vi "Curtin1_GlobalFolder.vi"() -> (1 "LabVIEW Data Path":path, 2 "Samples":path)   [LabVIEW 2022 SP3]
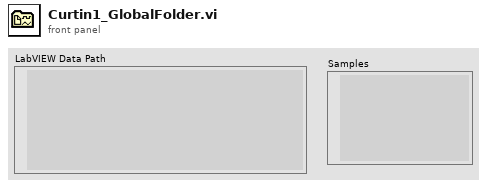
[diagram p1: front panel]
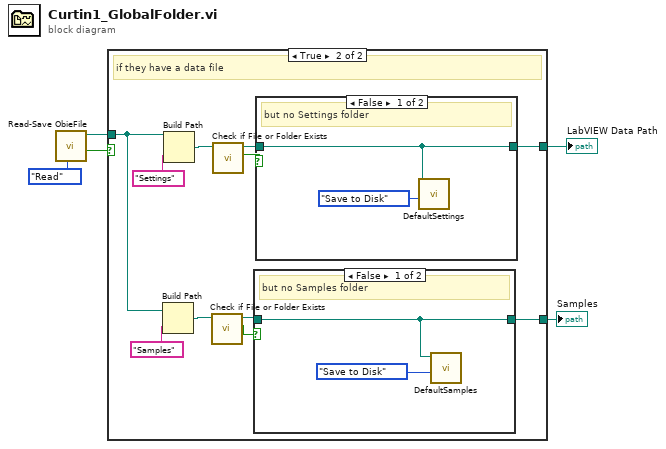
[diagram p0: block diagram]
diagram:
  n1 = call "Read-Save ObieFile.vi"("Task"=enum16{"Save", "Read"}."Read") -> ("Success?"=w2:bool, "DataPath Out"=w3:path)  [unwired: 8 in, 1 out]
  n2 = case shown="True" w2 {
    tunnel: [w6 w13] -> w5
    tunnel: w3 -> [w6 w10]
    tunnel: [w6 w7] -> w1
    frame False {
      # "they have not set up the data folder yet"
    }
    frame True {
      # "if they have a data file"
      n3 = Build Path(base path=w10, name or relative path="Samples") -> (appended path=w12:path)
      n4 = Build Path(base path=w10, name or relative path="Settings") -> (appended path=w14:path)
      n5 = call <vilib>:"Check if File or Folder Exists.vi"("path"=w12) -> ("file or folder exists?"=w8:bool, "dup path"=w9:path)  [unwired: 8 in, 1 out]
      n6 = call <vilib>:"Check if File or Folder Exists.vi"("path"=w14) -> ("file or folder exists?"=w16:bool, "dup path"=w15:path)  [unwired: 8 in, 1 out]
      n7 = case shown="False" w8 {
        tunnel: [w19 w20] -> w7
        tunnel: w9 -> [w19 w20]
        frame False {
          # "but no Samples folder"
          n8 = call "DefaultSamples.vi"("Task"=enum16{"Load to VI", "Save to Disk"}."Save to Disk", "path (use dialog)"=w19) -> ()  [unwired: 9 in, 1 out]
        }
        frame True {
          # "and a settings folder"
        }
      }
      n9 = case shown="False" w16 {
        tunnel: [w21 w23] -> w13
        tunnel: w15 -> [w21 w23]
        frame False {
          # "but no Settings folder"
          n10 = call "DefaultSettings.vi"("Task"=enum16{"Load to VI", "Save to Disk"}."Save to Disk", "path (use dialog)"=w21) -> ()  [unwired: 9 in, 1 out]
        }
        frame True {
          # "and a settings folder"
        }
      }
    }
  }
  "LabVIEW Data Path" <- w5
  "Samples" <- w1
